vi "MathOptim-Fit Power2.vi"(0 "Y":dbl[](array[numeric]), 5 "X":dbl[](array[numeric]), 11 "error in (no error)":errorcluster) -> (4 "best nonlinear fit":dbl[](array[numeric]), 6 "best fit parameters":dbl[](array[numeric]), 8 "SSE":dbl, 10 "adjusted R2":dbl, 13 "positive x":dbl[](array[numeric]), 14 "summary":string, 15 "error out":errorcluster)   [LabVIEW 2020]
uses:
  Array Manipulation VIs/Irregular Array Subset (DBL).vi
  <vilib>/gmath/NumericalOptimization/Nonlinear Curve Fit LM.vi
  <vilib>/gmath/NI_Gmath.lvlib
panel:
  out "R2":dbl
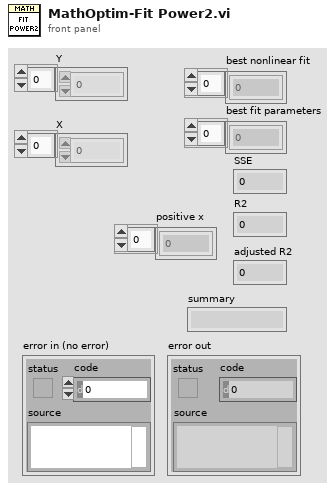
[diagram p1: front panel]
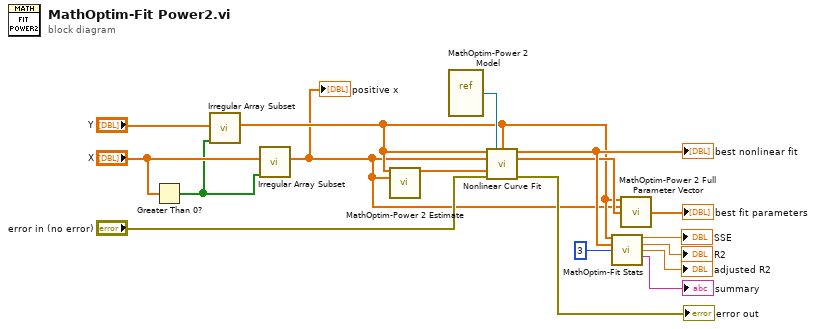
[diagram p0: block diagram]
diagram:
  n1 = Greater Than 0?(x="X") -> (x > 0?=w1:bool[])
  n2 = call-poly "Irregular Array Subset.vi"("Mask"=w1, "Array"="Y") -> ("Array Subset"=w4:dbl[])  [unwired: 8 in, 1 out]
  n3 = call-poly "Irregular Array Subset.vi"("Mask"=w1, "Array"="X") -> ("Array Subset"=w2:dbl[])  [unwired: 8 in, 1 out]
  "positive x" <- w2
  n4 = call "MathOptim-Power 2 Estimate.vi"("Y"=w4, "X"=w2) -> ("Initial guess"=w14:dbl[])  [unwired: 13 in]
  n5 = vi-ref "MathOptim-Power 2 Model.vi"() -> (w17:refnum<vi>)
  n6 = call-poly <vilib>:"Nonlinear Curve Fit.vi"("Y"=w4, "f(x,a)"=w17, "data"=w4, "X"=w2, "initial parameters"=w14, "error in (no error)"="error in (no error)") -> ("best nonlinear fit"=w8:dbl[], "best fit parameters"=w7:dbl[], "error out"=→"error out":errorcluster)  [unwired: 4 in, 3 out]
  "best nonlinear fit" <- w8
  n7 = call "MathOptim-Fit Stats.vi"("Y"=w4, "Yfit"=w8, "Num params"=3) -> ("SSE"=→"SSE":dbl, "R2"=→"R2":dbl, "adjusted R2"=→"adjusted R2":dbl, "summary"=→"summary":string)  [unwired: 9 in]
  n8 = call "MathOptim-Power 2 Full Parameter Vector.vi"("Y"=w4, "X"=w2, "a"=w7) -> ("parameters"=→"best fit parameters":dbl[])  [unwired: 12 in]
